vi "Publish Test Status.vi"(8 "error in (no error)":errorcluster, 11 "Model in":refnum<class "Model.lvclass">) -> (0 "error out":errorcluster, 3 "Model out":refnum<class "Model.lvclass">)   [LabVIEW 2016]
uses:
  User Events/User Events.lvclass
  Model.lvclass
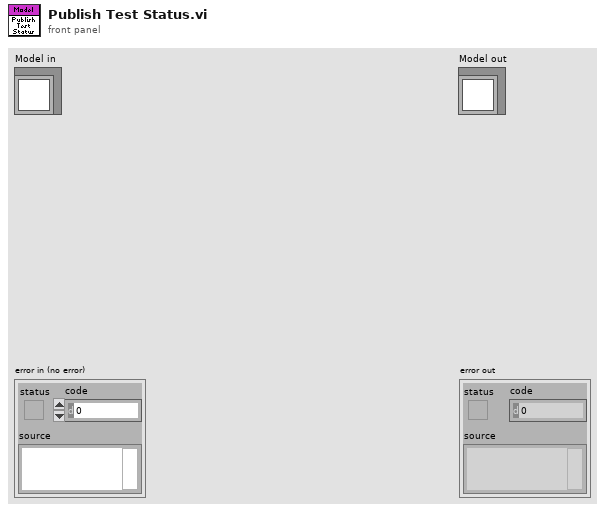
[diagram p1: front panel]
types:
  T1 = typedef "M1M3SupportEUI_TypeDefs.lvlib/Publish Data Events.ctl" = cluster{"State":refnum<user-event>, "ErrorCode":refnum<user-event>, "Scan Progress":refnum<user-event>, "All Test Status":refnum<user-event>}
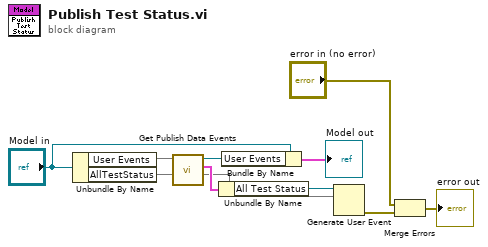
[diagram p0: block diagram]
diagram:
  n1 = Unbundle By Name("Model in") -> ("User Events"=w9, "AllTestStatus"=w6)
  n2 = call "Get Publish Data Events.vi"("UserEvents in"=w9) -> ("Publish Data Events"=w8:T1, "UserEvents out"=w5:refnum<class "User Events.lvclass">)  [unwired: 9 in]
  n3 = Unbundle By Name(w8) -> ("All Test Status"=w7:refnum<user-event>)
  n4 = Bundle By Name(cluster="Model in", "User Events"=w5) -> (→"Model out":cluster{})
  n5 = Generate User Event(user event=w7, event data cluster=w6) -> (error out=w4:errorcluster)  [unwired: 2 in, 1 out]
  n6 = Merge Errors("error in (no error)", w4) -> (→"error out":errorcluster)
